vi "Thev-Advance Procedure.vi"(0 "State in":T1, 5 "Params":T4 {"LProbe" items=["None"=-1, "Probe A"=0, "Probe B"=1]; "Rprobe" items=["None"=-1, "Probe A"=0, "Probe B"=1]}) -> (4 "State out":T1)   [LabVIEW 2015]
uses:
  Typedefs/Thev-Parameters.ctl
  Typedefs/Thev-Stimulus.ctl
  Typedefs/Thev-Find.ctl
  Misc VIs/Equipment Control/ER10X/ER10X-Probe.ctl
  Typedefs/Thev-State.ctl
  D:/Experiment VIs/Misc VIs/Equipment Control/ER10X/ER10XConnect.NET.dll
  Misc VIs/Equipment Control/ER10X/ER10XConnect.NET.dll
  Typedefs/Thev-Procedure Phase.ctl
  Typedefs/Thev-Progress Table Element.ctl
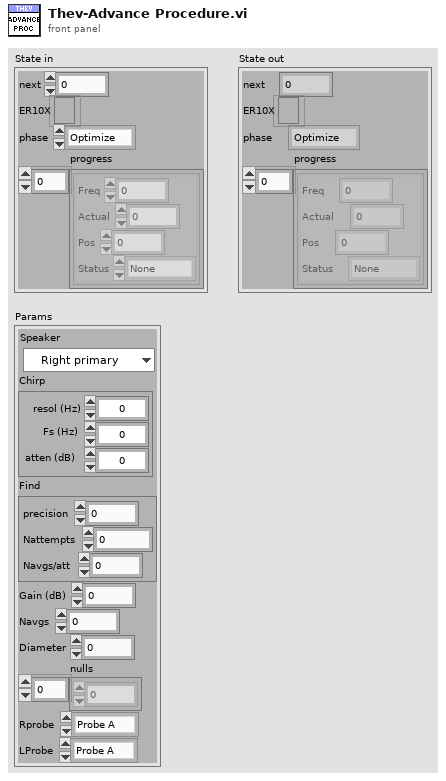
[diagram p1: front panel]
types:
  T1 = typedef "Thev-State.ctl" = cluster{"next":i32, "ER10X":refnum<k24>, "phase":T2, "progress":T3[]}
  T2 = typedef "Thev-Procedure Phase.ctl" = enum16{"Optimize", "Measure", "Compute", "Finished"}
  T3 = typedef "Thev-Progress Table Element.ctl" = cluster{"Freq":dbl, "Actual":dbl, "Pos":dbl, "Status":enum16{"None", "Measuring", "Finished"}}
  T4 = typedef "Thev-Parameters.ctl" = cluster{"Speaker":enum16{"Right primary", "Right secondary", "Left primary", "Left secondary"}, "Chirp":T5, "Find":T6, "Gain (dB)":dbl, "Navgs":i32, "Diameter":dbl, "nulls":dbl[], "Rprobe":T7, "LProbe":T7}
  T5 = typedef "Thev-Stimulus.ctl" = cluster{"resol (Hz)":dbl, "atten (dB)":dbl, "Fs (Hz)":dbl}
  T6 = typedef "Thev-Find.ctl" = cluster{"precision":dbl, "Nattempts":i32, "Navgs/att":i32}
  T7 = typedef "ER10X-Probe.ctl" = i32
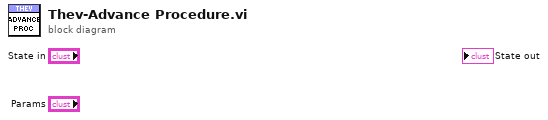
[diagram p0: block diagram]
diagram:
